vi "GenerateT1Mask.vi"(0 "Waveform":waveform(dbl)={"t0"=timestamp(0 s since 1904-01-01), "dt"=0.0, "Y"=[]}, 1 "Reset":bool, 5 "Polarity":bool, 11 "error in (no error)":errorcluster, 12 "Mask Selector":u16(ring)=1 items=["ITU", "EIA/TIA 547-1989"]) -> (4 "test passed?":bool, 6 "output values":waveform(dbl)[](array[waveform]), 15 "error out":errorcluster)   [LabVIEW 2012]
uses:
  <vilib>/measure/mamon.llb/Trigger Detection for 1 Channel (obs).vi
  <vilib>/measure/mamon.llb/Create Continuous Mask.vi
  Align Mask and Signal - cluster.vi
  <vilib>/measure/mamon.llb/Limit Testing Time.vi
  <vilib>/measure/NI_MAPro.lvlib
panel:
  in  "EIA/TIA Lower Specification Cluster":cluster{"ANSI X Low":dbl[], "ANSI Y Low":dbl[]}={"ANSI X Low"=[-3.238341e-07, -1.5e-07, -1.49e-07, -1e-07, 0.0, 1e-07, 1.49e-07, 1.5e-07, 3e-07, 4.25e-07], "ANSI Y Low"=[-0.05, -0.05, 0.5, 0.95, 0.95, 0.9, 0.5, -0.45, -0.45, -0.2]} {"ANSI Y Low" format="%.4e"; "ANSI X Low" format="%.4e"}
  in  "EIA/TIA Upper Specification Cluster":T1={"ANSI X High"=[-3.238341e-07, -2.5e-07, -1.75e-07, -1.74e-07, -7.5e-08, 0.0, 1.75e-07, 2.25e-07, 3.75e-07], "ANSI Y High"=[0.05, 0.05, 0.8, 1.15, 1.15, 1.05, 1.05, -0.07, 0.05]} {"ANSI Y High" format="%.4e"; "ANSI X High" format="%.4e"}
  in  "ITU Lower Specification Cluster":cluster{"ITU X Low":dbl[], "ITU Y Low":dbl[]}={"ITU X Low"=[-3.238341e-07, -1.36917e-07, -1.35917e-07, 0.0, 8.09585e-08, 1.35917e-07, 1.36917e-07, 2.158894e-07, 3.238341e-07], "ITU Y Low"=[-0.15, -0.15, 1.5, 2.3, 2.3, 1.5, -1.2, -1.2, -0.15]} {"ITU Y Low" format="%.2f"; "ITU X Low" format="%.4e"}
  in  "ITU Upper Specification Cluster":cluster{"ITU X High":dbl[], "ITU Y High":dbl[]}={"ITU X High"=[-3.238341e-07, -2.428756e-07, -1.86917e-07, -1.85917e-07, 1.85917e-07, 1.86917e-07, 2.428756e-07, 3.23834e-07], "ITU Y High"=[0.15, 0.15, 1.5, 3.7, 3.7, 1.5, 0.15, 0.15]} {"ITU Y High" format="%.2f"; "ITU X High" format="%.4e"}
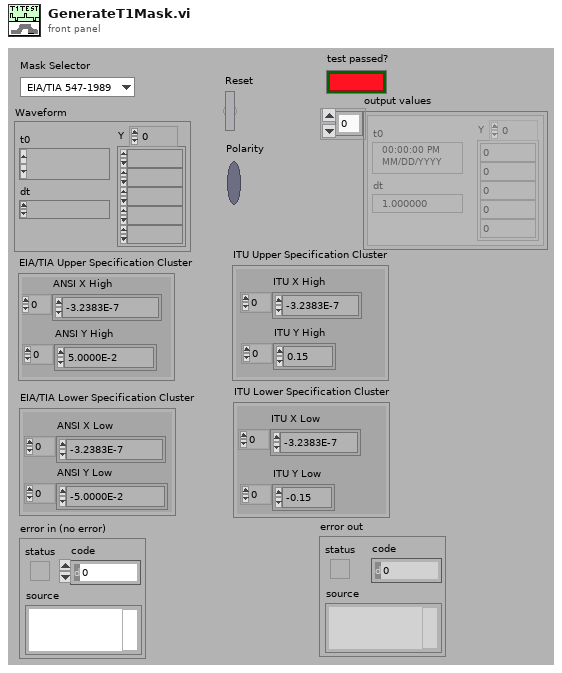
[diagram p1: front panel]
types:
  T1 = cluster{"ANSI X High":dbl[], "ANSI Y High":dbl[]}
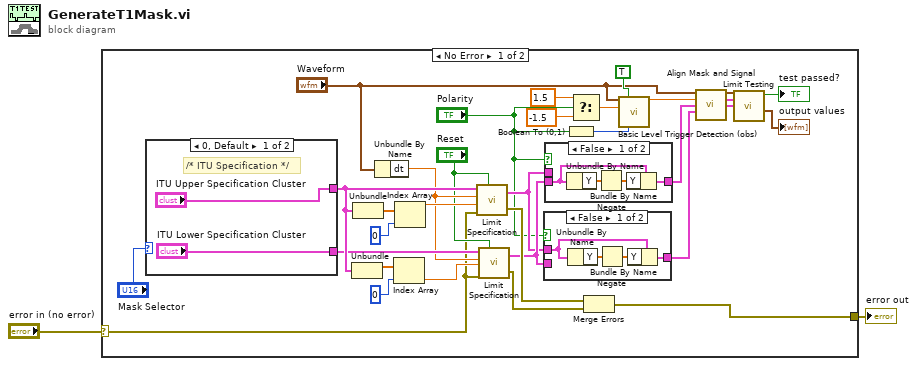
[diagram p0: block diagram]
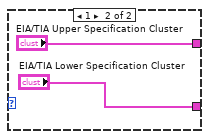
[diagram p4: hidden frame]
diagram:
  n1 = case shown="No Error" "error in (no error)" {
    selector: "error in (no error)" -> [w3 w49]
    tunnel: [w22 w49] -> w1
    frame No Error {
      n2 = case shown="0, Default" "Mask Selector" {
        tunnel: ["ITU Upper Specification Cluster" "EIA/TIA Upper Specification Cluster"] -> w27
        tunnel: ["ITU Lower Specification Cluster" "EIA/TIA Lower Specification Cluster"] -> w26
        frame 0, Default {
          # "/* ITU Specification */"
        }
        frame 1 {
        }
      }
      n3 = Unbundle(w27) -> ("ANSI X High"=w30:dbl[])  [unwired: 1 out]
      n4 = Unbundle(w27) -> ("ANSI X High"=w33:dbl[])  [unwired: 1 out]
      n5 = Unbundle By Name("Waveform") -> ("dt"=w23:dbl)
      n6 = Index Array(array=w30, index=0 ("Index")) -> (element=w28:dbl)
      n7 = Index Array(array=w33, index=0 ("Index")) -> (element=w31:dbl)
      n8 = call-poly <vilib>:"Limit Specification.vi"("Specification Cluster"=w27, "dx"=w23, "x0"=w31, "error in (no error)"=w3, "Reset"="Reset") -> ("Limit"=w19:cluster{"x0":dbl, "dx":dbl, "Y":dbl[]}, "error out"=w25:errorcluster)
      n9 = call-poly <vilib>:"Limit Specification.vi"("Specification Cluster"=w26, "dx"=w23, "x0"=w28, "error in (no error)"=w3, "Reset"="Reset") -> ("Limit"=w20:cluster{"x0":dbl, "dx":dbl, "Y":dbl[]}, "error out"=w24:errorcluster)
      n10 = case shown="False" "Polarity" {
        tunnel: w20 -> [_ w39]
        tunnel: [w35 w39] -> w9
        tunnel: w19 -> [w36 _]
        frame False {
          n11 = Unbundle By Name(w36) -> ("Y"=w38:dbl[])
          n12 = Negate(x=w38) -> (-x=w37:dbl[])
          n13 = Bundle By Name(cluster=w36, "Y"=w37) -> (w35:cluster{"x0":dbl, "dx":dbl, "Y":dbl[]})
        }
        frame True {
        }
      }
      n14 = case shown="False" "Polarity" {
        tunnel: [w40 w44] -> w10
        tunnel: w19 -> [_ w44]
        tunnel: w20 -> [w41 _]
        frame False {
          n15 = Unbundle By Name(w41) -> ("Y"=w42:dbl[])
          n16 = Negate(x=w42) -> (-x=w43:dbl[])
          n17 = Bundle By Name(cluster=w41, "Y"=w43) -> (w40:cluster{"x0":dbl, "dx":dbl, "Y":dbl[]})
        }
        frame True {
        }
      }
      n18 = Boolean To (0,1)(Boolean="Polarity") -> (0, 1=w17:i16)
      n19 = Select(t=1.5 ("level"), s="Polarity", f=-1.5 ("level")) -> (s? t:f=w13:dbl)
      n20 = Merge Errors(w25, w24) -> (w22:errorcluster)
      n21 = call-poly <vilib>:"Basic Level Trigger Detection (obs).vi"("signal in"="Waveform", "reset"=TRUE ("Reset"), "level"=w13, "trigger slope"=w17) -> ("trigger location"=w12:dbl)  [unwired: 9 in, 2 out]
      n22 = call-poly "Align Mask and Signal.vi"("Waveform"="Waveform", "trigger index"=w12, "upper limit"=w10, "lower limit"=w9) -> ("Waveform out"=w8:waveform(dbl), "upper limit out"=w7:cluster{"x0":dbl, "dx":dbl, "Y":dbl[]}, "lower limit out"=w6:cluster{"x0":dbl, "dx":dbl, "Y":dbl[]})  [unwired: 7 in, 2 out]
      n23 = call-poly <vilib>:"Limit Testing.vi"("lower limit"=w6, "upper limit"=w7, "signal in"=w8) -> ("output values"=→"output values":waveform(dbl)[], "test passed?"=→"test passed?":bool)  [unwired: 3 in, 4 out]
    }
    frame Error {
    }
  }
  "error out" <- w1
